vi "NET-RX Spawn TCP Service.vi"(4 "Stop Module":refnum<user-event>, 6 "Caller MsgQ":refnum<class "DQMH-GenNet Message Queue.lvclass">, 8 "error in":errorcluster, 9 "Module ID":i32=-1, 11 "Connection ID":refnum<k5>) -> (0 "error out":errorcluster)   [LabVIEW 2014, in "GenNet-Server.lvlib"]
doc: "Spawns a new TCP/IP service for a networked client. Sets <b>Connection ID</b> reference, <b>Module ID</b>, <b>Caller MsqQ</b> queue reference and <b>Stop Module</b> event reference before running the service VI."
uses:
  GenNet-Server.lvlib
  DQMH-GenNet Message Queue.lvclass
  Stop Argument--cluster.ctl
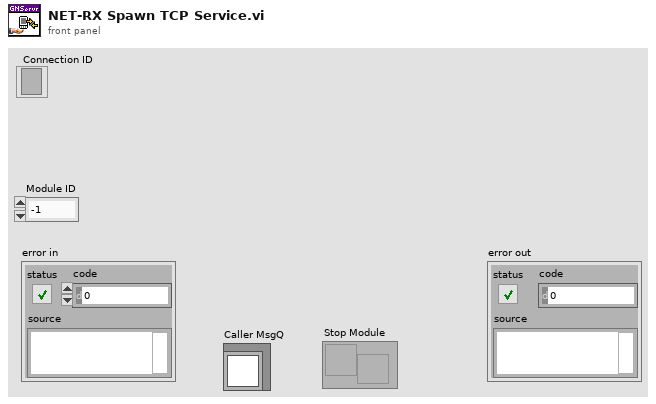
[diagram p1: front panel]
types:
  T1 = enum32{"Invalid", "Standard", "Closed", "Hidden", "Minimized", "Maximized"}
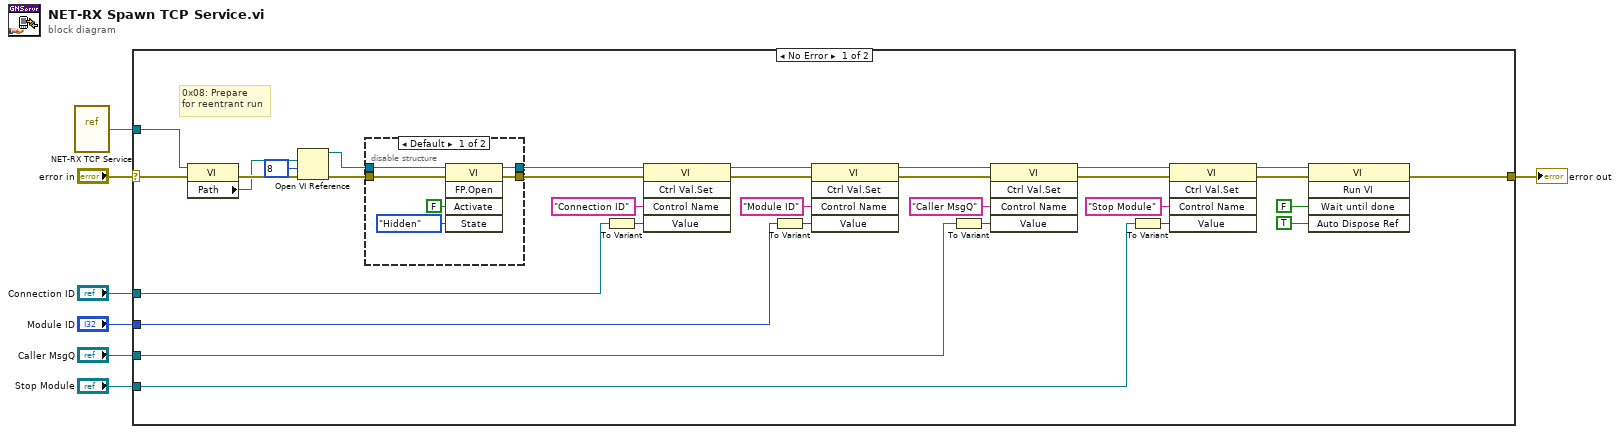
[diagram p0: block diagram]
diagram:
  n1 = vi-ref "NET-RX TCP Service.vi"() -> (w4:refnum<vi>)
  n2 = case shown="No Error" "error in" {
    selector: "error in" -> [w8 w46]
    tunnel: [w23 w46] -> w7
    tunnel: "Caller MsgQ" -> [w15 _]
    tunnel: "Module ID" -> [w14 _]
    tunnel: w4 -> [w13 _]
    tunnel: "Connection ID" -> [w12 _]
    tunnel: "Stop Module" -> [w9 _]
    frame No Error {
      # "0x08: Prepare \nfor reentrant run"
      n3 = property class="VI"(reference=w13, error in=w8) -> (error out=w30:errorcluster, "Path"=w29:path)  [unwired: 1 out]
      n4 = Open VI Reference(vi path=w29, options=8, error in (no error)=w30) -> (vi reference=w32:refnum<vi>, error out=w33:errorcluster)  [unwired: 3 in]
      n5 = disable-structure shown="Default" {
        disable-tunnel: [w43 w45] -> w28
        disable-tunnel: w33 -> [w42 w44]
        disable-tunnel: [w41 w44] -> w27
        disable-tunnel: w32 -> [w40 w45]
        frame condition #0 (active) {
          n6 = invoke class="VI" method="FP.Open"(reference=w40, error in=w42, "Activate"=FALSE ("Activate?"), "State"=T1."Hidden") -> (reference out=w43:refnum<vi>, error out=w41:errorcluster)  [unwired: 1 in, 3 out]
        }
        frame condition #1 {
        }
      }
      n7 = To Variant(anything=w12) -> (Variant=w34:variant)
      n8 = invoke class="VI" method="Ctrl Val.Set"(reference=w28, error in=w27, "Control Name"="Connection ID", "Value"=w34) -> (reference out=w20:refnum<vi>, error out=w19:errorcluster)  [unwired: 1 in, 3 out]
      n9 = To Variant(anything=w14) -> (Variant=w22:variant)
      n10 = invoke class="VI" method="Ctrl Val.Set"(reference=w20, error in=w19, "Control Name"="Module ID", "Value"=w22) -> (reference out=w18:refnum<vi>, error out=w17:errorcluster)  [unwired: 1 in, 3 out]
      n11 = To Variant(anything=w15) -> (Variant=w16:variant)
      n12 = invoke class="VI" method="Ctrl Val.Set"(reference=w18, error in=w17, "Control Name"="Caller MsgQ", "Value"=w16) -> (reference out=w25:refnum<vi>, error out=w24:errorcluster)  [unwired: 1 in, 3 out]
      n13 = To Variant(anything=w9) -> (Variant=w11:variant)
      n14 = invoke class="VI" method="Ctrl Val.Set"("Control Name"="Stop Module", "Value"=w11) -> ()  [unwired: 3 in, 5 out]
      n15 = invoke class="VI" method="Run VI"(reference=w25, error in=w24, "Wait until done"=FALSE ("Wait Until Done"), "Auto Dispose Ref"=TRUE ("Auto Dispose Reference")) -> (error out=w23:errorcluster)  [unwired: 1 in, 4 out]
    }
    frame Error {
    }
  }
  "error out" <- w7
